vi "XML Get Actuation Chassis.vi"(11 "Actuation Network":T2) -> (1 "Actuation Chassis Names":string[](array[string]), 2 "Number of Correctors":i32, 3 "Actuation Variable Names":string[][](array[string]), 4 "Inverse PS Matrix Mapping":u32[][](array[numeric]), 5 "PS Parameters":T1[](array[typedef]), 6 "PS Matrix Mapping":cluster{u32[]}[](array[cluster]), 7 "Selected Correctors":u32[](array[numeric]))   [LabVIEW 2011, in "XML VIs.lvlib"]
doc: "Extracts the Actuation Network configuration data (ordered by chassis) and builds dedicated clusters for each configuration (ordered by response matrix column indexes).\nThe \"PS Matrix Mapping\" is used to decode the digital I/O of all Actuation Chassis to byte words representing each chasiss digital I/Os (each bit comes from one of the 8 chassis actuators) to a vector of boolean values in the response matrix column indexes order. \nThe \"Inverse PS Matrix Mapping\" is used to encode the digital I/O of all Actuation Chassis from a vector of boolean values in the response matrix column indexes order to byte words representing each chasiss digital I/Os (each bit comes from one of the 8 chassis actuators)."
uses:
  XML VIs.lvlib
  Types Definitions/Type Actuation Network Configuration.ctl
  Types Definitions/Type PS Parameters.ctl
  Type Definitions.lvlib
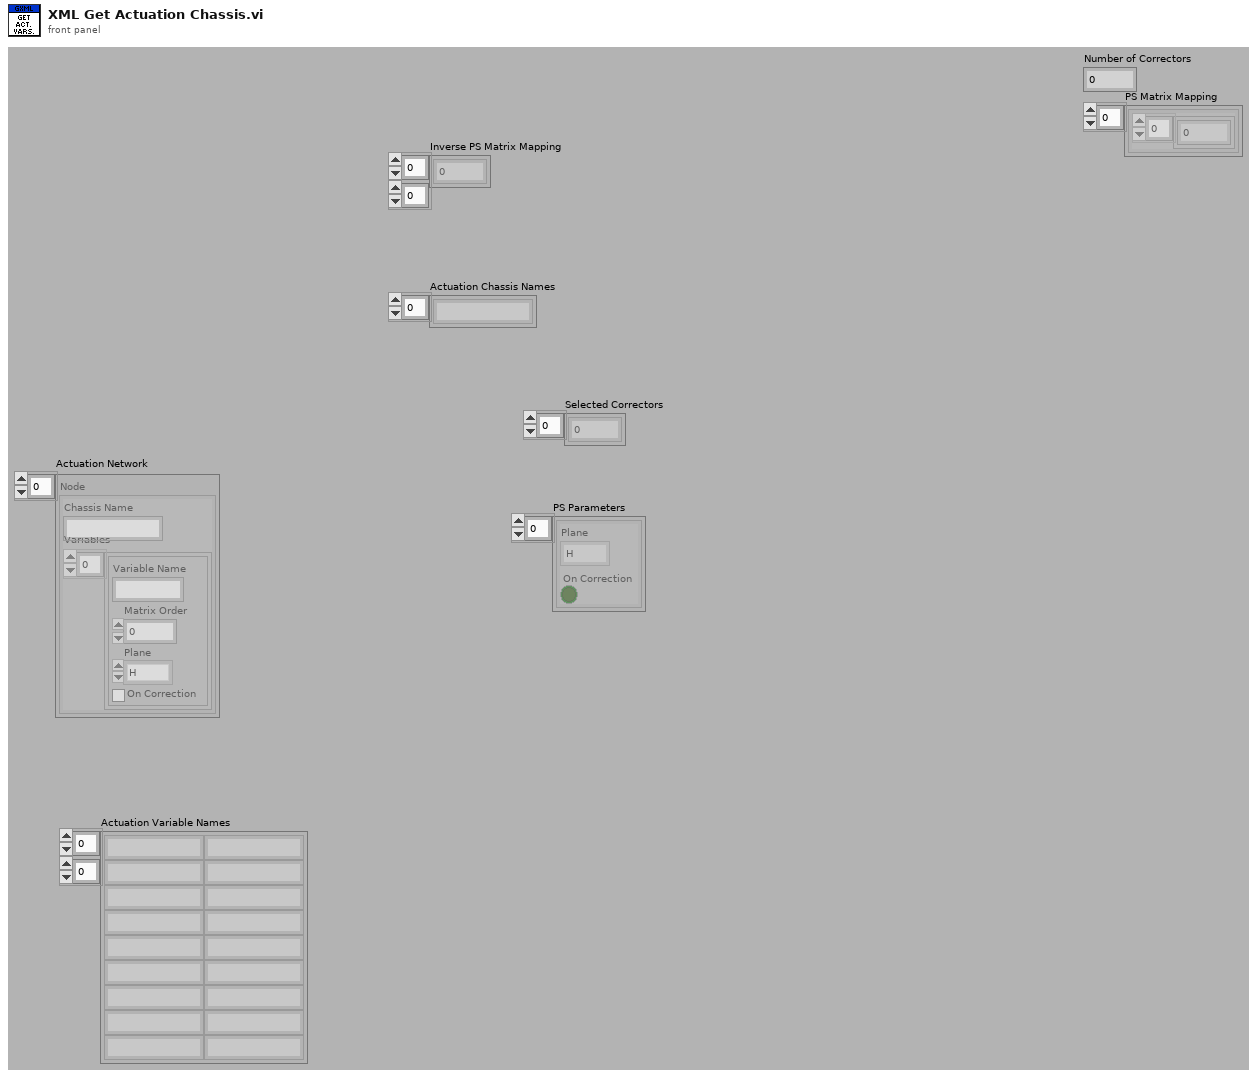
[diagram p1: front panel]
types:
  T1 = typedef "Type Definitions.lvlib/Type PS Parameters.ctl" = cluster{"Plane":enum8{"H", "V"}, "On Correction":bool}
  T2 = typedef "Type Definitions.lvlib/Type Actuation Network Configuration.ctl" = cluster{"Chassis Name":string, "Variables":cluster{"Variable Name":string, "Matrix Order":u32, "Plane":enum8{"H", "V"}, "On Correction":bool}[]}[]
  T3 = cluster{"Variable Name":string, "Matrix Order":u32, "Plane":enum8{"H", "V"}, "On Correction":bool}[]
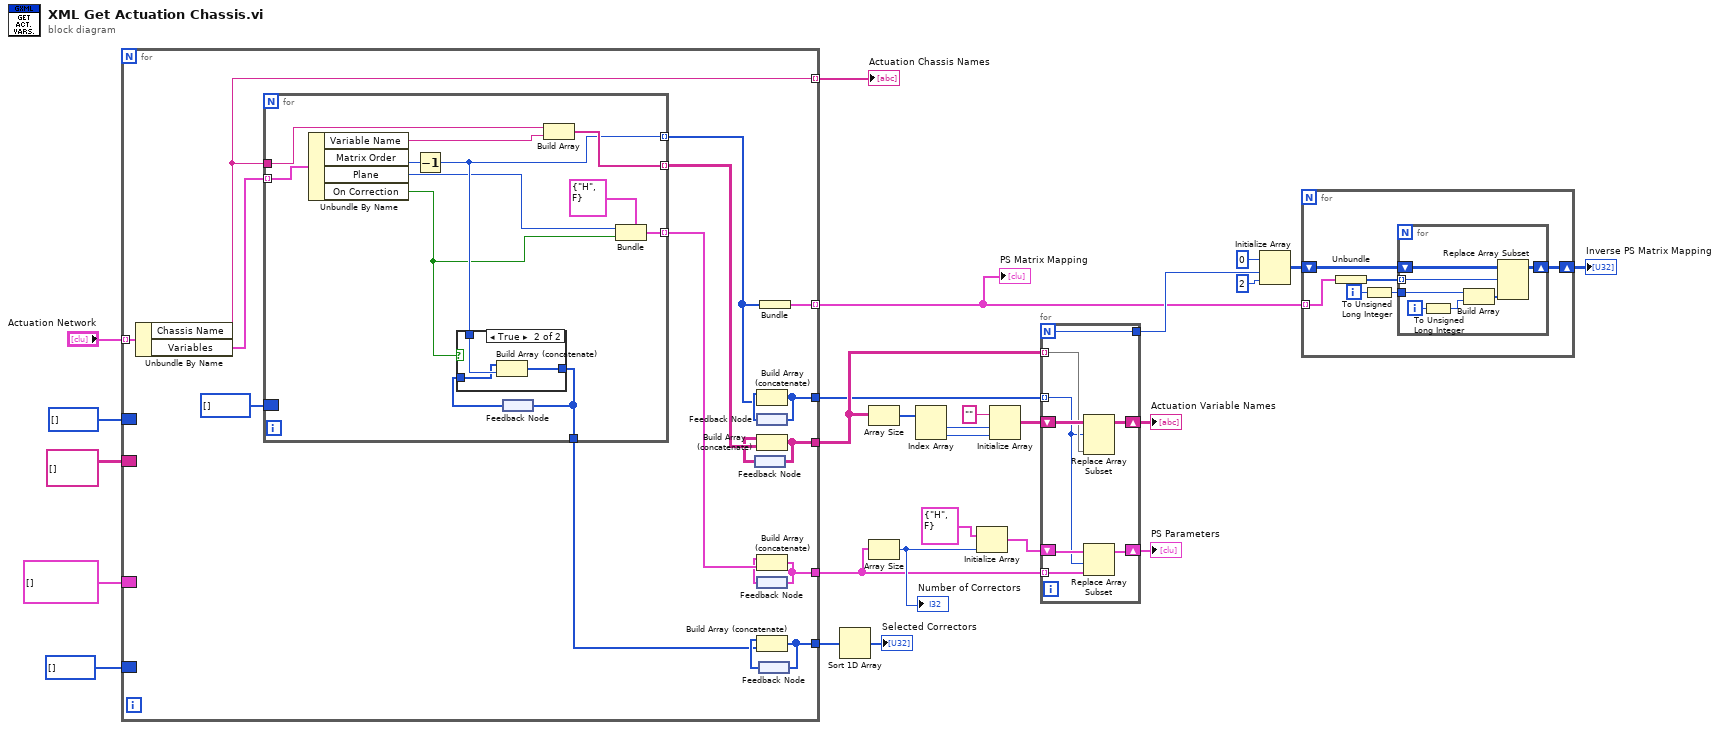
[diagram p0: block diagram]
diagram:
  n1 = for {
    tunnel: "Actuation Network" -> [w44] mode=indexing
    tunnel: [w39] -> w19 mode=indexing
    border: T1[] [] -> [_]
    tunnel: [w36] -> w1
    border: string[][] [] -> [_]
    tunnel: [w35] -> w7
    border: u32[] [] -> [_]
    tunnel: [w34] -> w6
    border: u32[] [] -> [_]
    tunnel: [w32] -> w4
    tunnel: [w28] -> w2 mode=indexing
    n2 = Unbundle By Name(w44) -> ("Chassis Name"=w39:string, "Variables"=w43:T3)
    n3 = for {
      tunnel: w43 -> [w56] mode=indexing
      tunnel: w39 -> [w54]
      tunnel: [w49] -> w29 mode=indexing
      tunnel: [w53] -> w42 mode=indexing
      tunnel: [w51] -> w38 mode=indexing
      border: u32[] [] -> [_]
      tunnel: [w47] -> w30
      n4 = Unbundle By Name(w56) -> ("Variable Name"=w55:string, "Matrix Order"=w52:u32, "Plane"=w46:enum8{"H", "V"}, "On Correction"=w45:bool)
      n5 = Decrement(x=w52) -> (x-1=w49:u32)
      n6 = feedback #1() -> (w48:u32[])
      n7 = case shown="True" w45 {
        tunnel: w49 -> [_ w60]
        tunnel: w48 -> [w57 w59]
        tunnel: [w57 w58] -> w47
        frame False {
        }
        frame True {
          n8 = Build Array (concatenate)(w59, w60) -> (w58:u32[])
        }
      }
      n9 = feedback-in #1(w47) -> ()
      n10 = Build Array(w54, w55) -> (w53:string[])
      n11 = Bundle(cluster=T1 {"Plane"=enum."H", "On Correction"=FALSE}, "Plane"=w46, "On Correction"=w45) -> (w51:T1)
    }
    n12 = feedback #2() -> (w41:string[][])
    n13 = feedback #3() -> (w40:u32[])
    n14 = Build Array (concatenate)(w40, w29) -> (w34:u32[])
    n15 = feedback-in #3(w34) -> ()
    n16 = Build Array (concatenate)(w41, w42) -> (w35:string[][])
    n17 = feedback-in #2(w35) -> ()
    n18 = feedback #4() -> (w37:T1[])
    n19 = Build Array (concatenate)(w37, w38) -> (w36:T1[])
    n20 = feedback-in #4(w36) -> ()
    n21 = feedback #5() -> (w31:u32[])
    n22 = Build Array (concatenate)(w31, w30) -> (w32:u32[])
    n23 = feedback-in #5(w32) -> ()
    n24 = Bundle(w29) -> (w28:cluster{u32[]})  [unwired: 1 in]
  }
  "Actuation Chassis Names" <- w19
  "PS Matrix Mapping" <- w2
  n25 = Sort 1D Array(array=w4) -> (sorted array=→"Selected Correctors":u32[])
  n26 = Array Size(array=w7) -> (size(s)=w25:i32[])
  n27 = Array Size(array=w1) -> (size(s)=w12:i32)
  "Number of Correctors" <- w12
  n28 = Index Array(array=w25) -> (element #1=w24:i32, element #2=w23:i32)  [unwired: 2 in]
  n29 = Initialize Array(T1 {"Plane"=enum."H", "On Correction"=FALSE} ("cluster"), w12) -> (w11:T1[])
  n30 = Initialize Array("" ("element"), w24, w23) -> (w22:string[][])
  n31 = for {
    N -> [w65]
    tunnel: w7 -> [w66] mode=indexing
    tunnel: w6 -> [w61] mode=indexing
    shift-right: [w67] -> w21
    shift-left: w22 -> [w68]
    tunnel: [w65] -> w13
    tunnel: w1 -> [w62] mode=indexing
    shift-right: [w63] -> w8
    shift-left: w11 -> [w64]
    n32 = Replace Array Subset(array=w68, new element=w66, index (row)=w61) -> (w67:string[][])  [unwired: 1 in]
    n33 = Replace Array Subset(array=w64, new element=w62, index=w61) -> (w63:T1[])
  }
  "Actuation Variable Names" <- w21
  "PS Parameters" <- w8
  n34 = Initialize Array(u32 0 ("element"), w13, 2 ("dimension size")) -> (w15:u32[][])
  n35 = for {
    shift-right: [w73] -> w14
    shift-left: w15 -> [w74]
    tunnel: w2 -> [w70] mode=indexing
    i -> [w72]
    n36 = Unbundle(w70) -> (w69:u32[])
    n37 = To Unsigned Long Integer(number=w72) -> (unsigned 32bit integer=w71:u32)
    n38 = for {
      tunnel: w71 -> [w79]
      shift-right: [w80] -> w73
      shift-left: w74 -> [w81]
      tunnel: w69 -> [w75] mode=indexing
      i -> [w76]
      n39 = To Unsigned Long Integer(number=w76) -> (unsigned 32bit integer=w77:u32)
      n40 = Build Array(w79, w77) -> (w78:u32[])
      n41 = Replace Array Subset(array=w81, new element=w78, index (row)=w75) -> (w80:u32[][])  [unwired: 1 in]
    }
  }
  "Inverse PS Matrix Mapping" <- w14
